vi "SPI Engine. Main.vi"(8 "error in":errorcluster, 10 "SPI Read Data":T3, 11 "SPI API References":T2={"DLU To SPI Engine Data FIFO"="DLU To SPI Engine Data", "SPI Engine to DLU Data FIFO"="SPI Engine to DLU Data", "Data to SPI Engine (Cache) Register"="Data to SPI Engine (Cache)", "SPI Settings to SPI Engine (Cache) Register"="SPI PHY Settings to SPI Engine (Cache)"}) -> (0 "error out":errorcluster, 1 "Chip Select ID":u8, 2 "SPI DIO Output":T4, 3 "SPI API References Out":T2={"DLU To SPI Engine Data FIFO"="DLU To SPI Engine Data", "SPI Engine to DLU Data FIFO"="SPI Engine to DLU Data", "Data to SPI Engine (Cache) Register"="Data to SPI Engine (Cache)", "SPI Settings to SPI Engine (Cache) Register"="SPI PHY Settings to SPI Engine (Cache)"})   [LabVIEW 2015]
doc: "This VI is the actual SPI Engine. It handles the SPI communication to the SPI bus."
uses:
  <userlib>/_NI SPI IP/FPGA/Controllers/Public/Spi Master Outputs.ctl
  <userlib>/_NI SPI IP/FPGA/Controllers/Public/Spi Master Inputs.ctl
  Controls/SPI API References.ctl
  Controls/SPI API Response Data.ctl
  <userlib>/_NI SPI IP/FPGA/Controllers/NI SPI IP FPGA.lvlib
panel:
  out "Output Data":T1
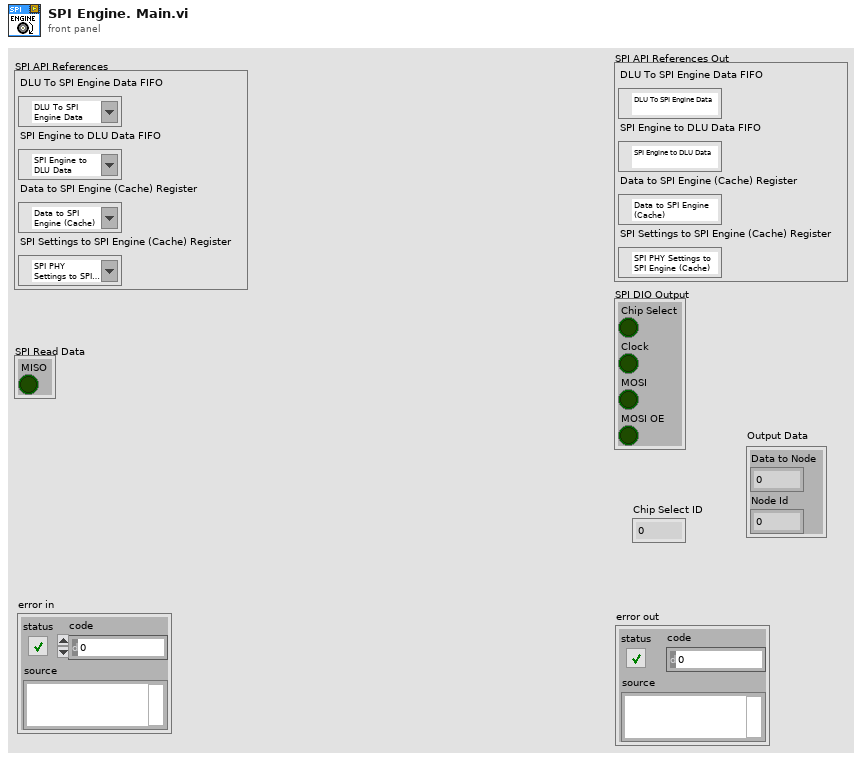
[diagram p1: front panel]
types:
  T1 = typedef "SPI API Response Data.ctl" = cluster{"Data to Node":u64, "Node Id":u16}
  T2 = typedef "SPI API References.ctl" = cluster{"DLU To SPI Engine Data FIFO":refnum<k21>, "SPI Engine to DLU Data FIFO":refnum<k21>, "Data to SPI Engine (Cache) Register":refnum<k21>, "SPI Settings to SPI Engine (Cache) Register":refnum<k21>}
  T3 = typedef "NI SPI IP FPGA.lvlib/Spi Master Inputs.ctl" = cluster{"MISO":bool}
  T4 = typedef "NI SPI IP FPGA.lvlib/Spi Master Outputs.ctl" = cluster{"Chip Select":bool, "Clock":bool, "MOSI":bool, "MOSI OE":bool}
  T5 = typedef "SPI API Transaction Packet.ctl" = cluster{"Chip Select ID":u8, "SPI Data":u64, "Start Strobe":bool, "SPI Physical Settings":cluster{"Divide Value":u8, "Transfer Length (bits)":u8, "CS Asserted Polarity":bool, "Clock Polarity (CPOL)":bool, "Clock Phase (CPHA)":bool, "Lengthen MISO Setup":bool, "Direction Change Bit":u8, "MOSI Starts as Output":bool, "Tristatable MOSI":bool}}
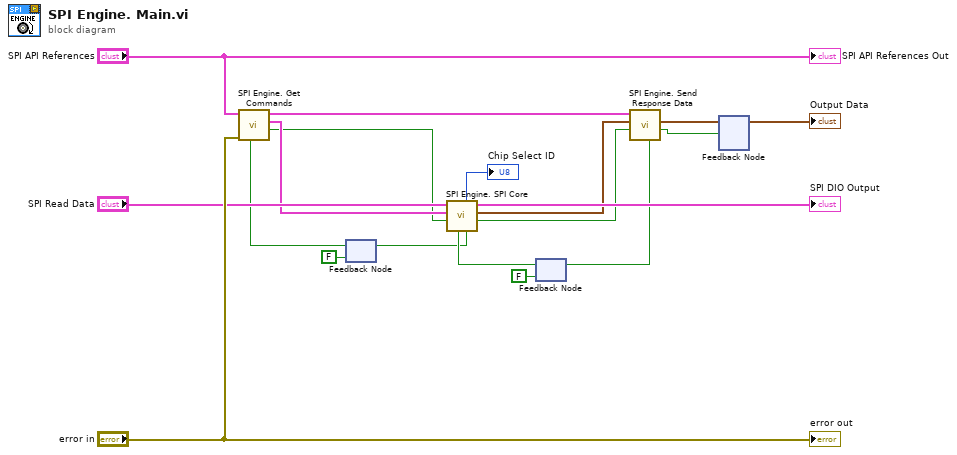
[diagram p0: block diagram]
diagram:
  n1 = feedback #1(FALSE ("ready for input")) -> (w16:bool)
  n2 = call "SPI Engine. Get Commands.vi"("Ready for Output"=w16, "error in"="error in", "Private Data In"="SPI API References") -> ("Output Valid"=w7:bool, "SPI Transaction Packet"=w8:T5, "Private Data Out"=w15:T2)  [unwired: 4 in, 2 out]
  n3 = feedback #2(FALSE ("Ready for Input")) -> (w14:bool)
  n4 = call "SPI Engine. SPI Core.vi"("Ready for Output"=w14, "Input Valid"=w7, "SPI Information In"=w8, "SPI DIO Input"="SPI Read Data") -> ("Output Valid"=w5:bool, "SPI Output Data"=w2:T1, "SPI DIO Output"=→"SPI DIO Output":T4, "Ready For Input"=w11:bool, "Chip Select ID"=→"Chip Select ID":u8)  [unwired: 3 in]
  n5 = feedback-in #1(w11) -> ()
  n6 = call "SPI Engine. Send Response Data.vi"("Input Valid"=w5, "Input Data"=w2, "Private Data In"=w15) -> ("New Data Sent?"=w6:bool, "Output Data"=w9:T1, "Ready for Input"=w13:bool)  [unwired: 5 in, 1 out]
  n7 = feedback-in #2(w13) -> ()
  n8 = feedback-in #3(w9, w6) -> ()
  n9 = feedback #3() -> (→"Output Data":T1)  [unwired: 1 in]
  "error out" <- "error in"
  "SPI API References Out" <- "SPI API References"
